vi "DFD I16 to FXP (scalar).vi"(7 "quantization settings":T1={"source"=0, "wl"=16, "iwl"=1, "overflow mode"=enum."Wrap", "rounding mode"=enum."Truncation", "signed?"=TRUE} {"source" items=["Coefficients a/k"=0, "Coefficients b/v"=7, "Input"=1, "Output"=2, "Multiplicand"=3, "Product"=4, "Sum"=5, "Delay"=6]}, 8 "error in (no error)":errorcluster, 11 "I16":i16) -> (0 "error out":errorcluster, 3 "FXP value":dbl)   [LabVIEW 2017, in "NI_DigFilterLicensed.lvlib"]
doc: "Converts integers to fixed-point numbers. Wire data to the <B>I16</B> input to determine the polymorphic instance to use or manually select the instance."
uses:
  <vilib>/addons/Digital Filter Design/NI_DigFilterLicensed.lvlib
  <vilib>/addons/Digital Filter Design/_Objects.llb/DFD Quantization Settings.ctl
  <vilib>/addons/Digital Filter Design/_Objects.llb/DFD Quantization Sources.ctl
  <vilib>/addons/Digital Filter Design/FXPLib.llb/dfd_FXP Casting (scaler).vi
  <vilib>/addons/Digital Filter Design/NI_DigFilter_FXP.lvlib
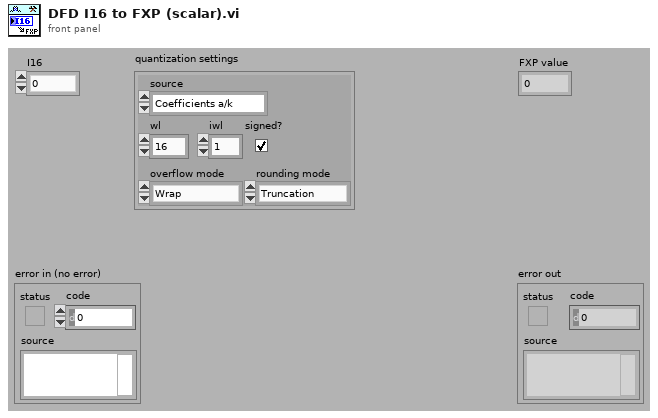
[diagram p1: front panel]
types:
  T1 = typedef "NI_DigFilterLicensed.lvlib/DFD Quantization Settings.ctl" = cluster{"source":T2, "wl":i16, "iwl":i16, "overflow mode":enum16{"Saturation", "Wrap"}, "rounding mode":enum16{"Nearest", "Truncation"}, "signed?":bool}
  T2 = typedef "NI_DigFilterLicensed.lvlib/DFD Quantization Sources.ctl" = u16
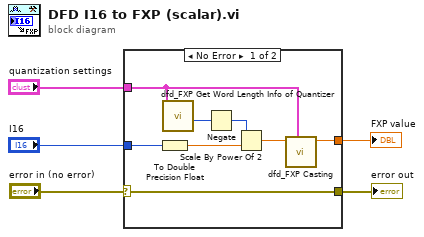
[diagram p0: block diagram]
diagram:
  n1 = case shown="No Error" "error in (no error)" {
    selector: "error in (no error)" -> [w6 w14]
    tunnel: "I16" -> [w12 _]
    tunnel: [w11 _] -> w4
    tunnel: "quantization settings" -> [w10 _]
    tunnel: [w6 w14] -> w1
    frame No Error {
      n2 = To Double Precision Float(number=w12) -> (double precision float=w9:dbl)
      n3 = call <vilib>:"dfd_FXP Get Word Length Info of Quantizer.vi"("quantization settings"=w10) -> ("fwl"=w13:i16)  [unwired: 10 out]
      n4 = Negate(x=w13) -> (-x=w8:i16)
      n5 = Scale By Power Of 2(n=w8, x=w9) -> (x*2^n=w7:dbl)
      n6 = call-poly <vilib>:"dfd_FXP Casting.vi"("quantization settings"=w10, "value in"=w7) -> ("value out"=w11:dbl)  [unwired: 1 in, 6 out]
    }
    frame Error {
    }
  }
  "FXP value" <- w4
  "error out" <- w1
